vi "uiControlsMgr.vi"(8 "error in (no error)":errorcluster, 9 "Captions File":string, 11 "VI reference":refnum<vi>) -> (0 "error out":errorcluster, 3 "uiControlsMgr out":refnum<class "uiControlsMgr.lvclass">)   [LabVIEW 2020, in "uiControlsMgr.lvclass"]
uses:
  uiControlsMgr.lvclass
  uiControlsMgr.lvclass/uiControlsMgr.ctl
  <vilib>/Utility/file.llb/Read Delimited Spreadsheet (string).vi
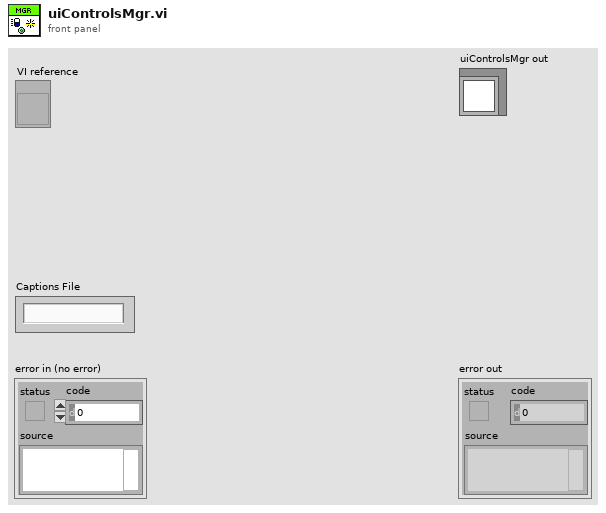
[diagram p1: front panel]
types:
  T1 = cluster{"Caption":string, "Ctl Refnum":refnum<vi>}
  T2 = map{string, cluster{"Caption":string, "Ctl Refnum":refnum<vi>}}
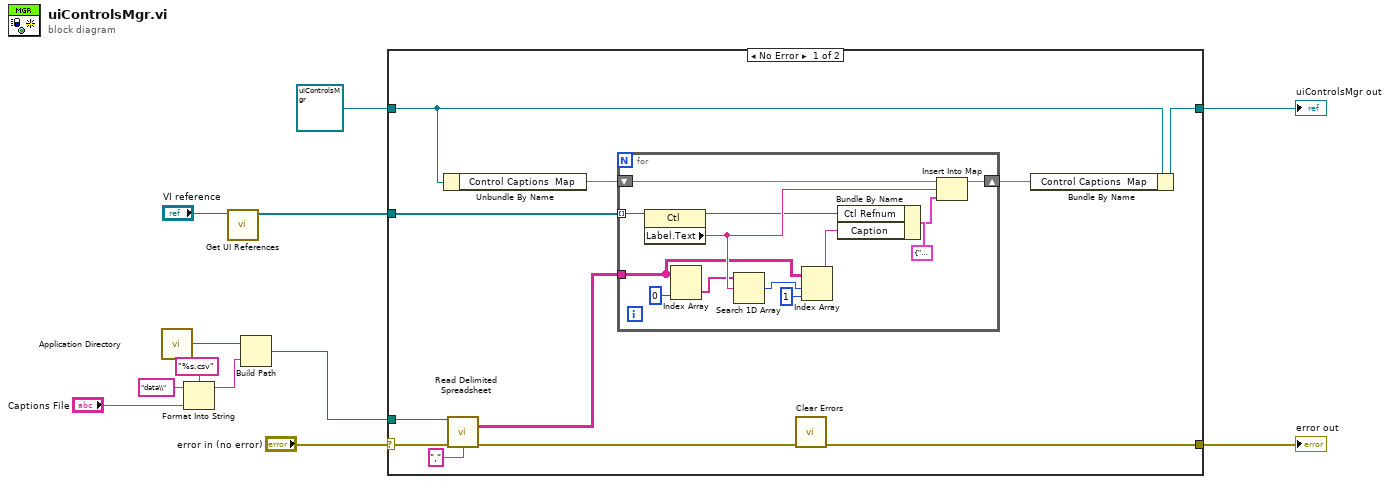
[diagram p0: block diagram]
diagram:
  n1 = call <vilib>:"Application Directory.vi"() -> ("Application Directory"=w8:path)
  n2 = Format Into String(format string="%s.csv", initial string="data\\", "Captions File") -> (resulting string=w4:string)  [unwired: 1 in, 1 out]
  n3 = call "Get UI References.vi"("VI reference"="VI reference") -> ("Controls[]"=w2:refnum<vi>[])  [unwired: 9 in, 1 out]
  n4 = Build Path(base path=w8, name or relative path=w4) -> (appended path=w3:path)
  n5 = case shown="No Error" "error in (no error)" {
    selector: "error in (no error)" -> [w23 w38]
    tunnel: [w13 w38] -> w11
    tunnel: [w20 w37] -> w9
    tunnel: refnum<class "uiControlsMgr.lvclass"> refnum ("uiControlsMgr in") -> [w22 w37]
    tunnel: w2 -> [w14 _]
    tunnel: w3 -> [w17 _]
    frame No Error {
      n6 = Unbundle By Name(w22) -> ("Control Captions  Map"=w21:T2)
      n7 = call-poly <vilib>:"Read Delimited Spreadsheet.vi"("file path (dialog if empty)"=w17, "error in (no error)"=w23, "delimiter (\\t)"="," ("delimiter (\\t)")) -> ("all rows"=w15:string[][], "error out"=w18:errorcluster)  [unwired: 7 in, 4 out]
      n8 = for {
        tunnel: w14 -> [w34] mode=indexing
        shift-right: [w35] -> w19
        shift-left: w21 -> [w36]
        tunnel: w15 -> [w29]
        n9 = property class="Ctl"(reference=w34) -> (reference out=w25:refnum<vi>, "Label.Text"=w33:string)  [unwired: 1 in, 1 out]
        n10 = Index Array(array=w29, index (col)=0 ("disabled index (col)")) -> (element=w31:string[])  [unwired: 1 in]
        n11 = Search 1D Array(1D array=w31, element=w33) -> (index of element=w28:i32)  [unwired: 1 in]
        n12 = Index Array(array=w29, index (row)=w28, index (col)=1 ("disabled index (col)")) -> (element=w24:string)
        n13 = Bundle By Name(cluster=T1 {"Caption"="", "Ctl Refnum"=refnum} ("Control Data"), "Ctl Refnum"=w25, "Caption"=w24) -> (w26:T1)
        n14 = Insert Into Map(map in=w36, key=w33, value=w26) -> (map out=w35:T2)  [unwired: 2 out]
      }
      n15 = call <vilib>:"Clear Errors.vi"("error in (no error)"=w18) -> ("error out"=w13:errorcluster)  [unwired: 5 in, 1 out]
      n16 = Bundle By Name(cluster=w22, "Control Captions  Map"=w19) -> (w20:refnum<class "uiControlsMgr.lvclass">)
    }
    frame Error {
    }
  }
  "error out" <- w11
  "uiControlsMgr out" <- w9
